vi "MainGui-Reboot.vi"(8 "error in (no error)":errorcluster) -> (0 "error out":errorcluster)   [LabVIEW 2016]
uses:
  MainGui.Action.ctl
  Global/ApplicationGlobal.vi
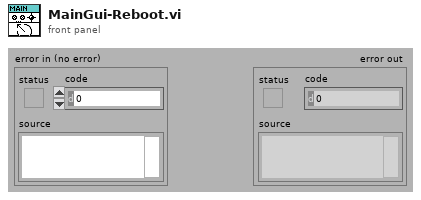
[diagram p1: front panel]
types:
  T1 = typedef "MainGui.Action.ctl" = enum32{"idle", "constructor", "destructor", "--- MainGui ---", "Gui.Translate", "Error.Update", "Error.Confirm", "TopBar.Update", "Buttons.Update", "StatusMsg.Update", "StatusTable.Update", "LogsTable.Update", "PLCReasemblyDone"}
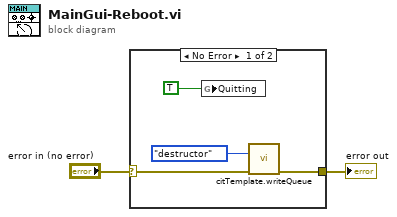
[diagram p0: block diagram]
diagram:
  n1 = case shown="No Error" "error in (no error)" {
    selector: "error in (no error)" -> [w3 w7]
    tunnel: [w6 w7] -> w1
    frame No Error {
      n2 = global write "ApplicationGlobal.vi" "Quitting"(TRUE ("Quitting")) -> ()
      n3 = call "citTemplate.writeQueue.vi"("event in (if not connected:all statemachine with data event)"=MainGui.Action."destructor" ("Action"), "error in (no error)"=w3) -> ("error out"=w6:errorcluster)  [unwired: 13 in]
    }
    frame Error {
    }
  }
  "error out" <- w1
